vi "8FFTHanning窗校正子程序.vi"(6 "averaging parameters":T1={"averaging mode"=enum."No averaging", "weighting mode"=enum."Exponential", "number of averages"=10}, 7 "time signal":waveform(dbl) caption="时间信号") -> (0 "FFT幅值":cluster{"f0":dbl, "df":dbl, "magnitude":dbl[]}(graph), 2 "FFT相位":cluster{"f0":dbl, "df":dbl, "phase":dbl[]}(graph), 3 "频率":dbl)   [LabVIEW 2017]
uses:
  <vilib>/Analysis/4window.llb/windowTd.ctl
  <vilib>/measure/maspectr.llb/FFT Spectrum (Mag-Phase) for 1 Chan.vi
  <vilib>/measure/NI_MAPro.lvlib
  <vilib>/Analysis/NI_AALPro.lvlib
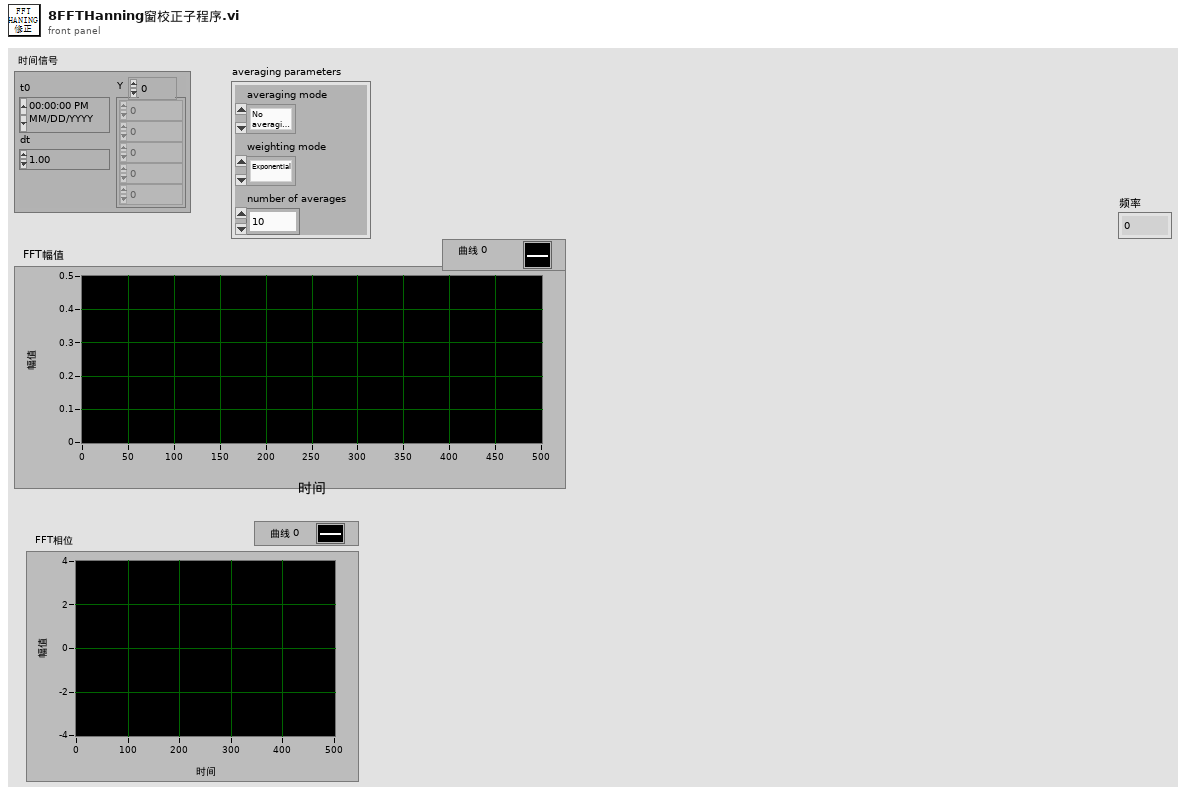
[diagram p1: front panel]
types:
  T1 = cluster{"averaging mode":enum16{"No averaging", "Vector averaging", "RMS averaging", "Peak hold"}, "weighting mode":enum16{"Linear", "Exponential"}, "number of averages":u32}
  T2 = typedef "NI_AALPro.lvlib/windowTd.ctl" = u32
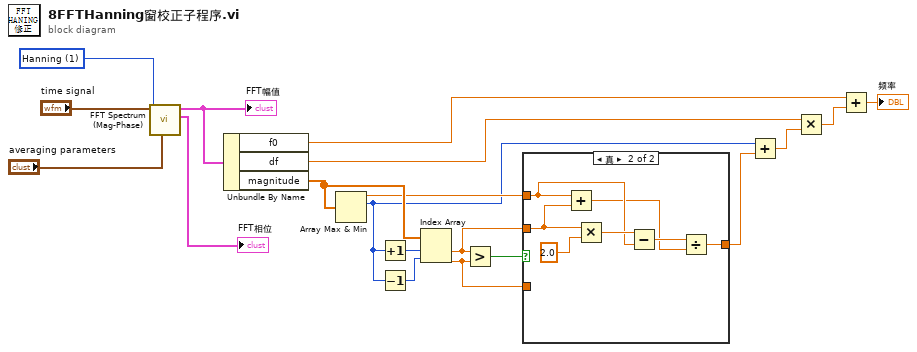
[diagram p0: block diagram]
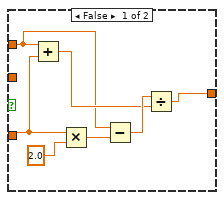
[diagram p2: hidden frame]
diagram:
  w17 = T2 1 items=["矩形"=0, "Hanning"=1, "Hamming"=2, "Blackman-Harris"=3, "Exact Blackman"=4, "Blackman"=5, "Flat Top"=6, "4阶Blackman-Harris "=7, "7阶Blackman-Harris"=8, "Low Sidelobe"=9, "Blackman Nuttall"=11, "三角"=30, "Bartlett-Hanning"=31, "Bohman"=32, "Parzen"=33, "Welch"=34, "Kaiser"=60, "Dolph-Chebyshev"=61, "高斯"=62] ("window")
  n1 = call-poly <vilib>:"FFT Spectrum (Mag-Phase).vi"("averaging parameters"="averaging parameters", "window"=w17, "time signal"="time signal") -> ("phase"=→"FFT相位":cluster{"f0":dbl, "df":dbl, "phase":dbl[]}, "magnitude"=w19:cluster{"f0":dbl, "df":dbl, "magnitude":dbl[]})  [unwired: 4 in, 3 out]
  "FFT幅值" <- w19
  n2 = Unbundle By Name(w19) -> ("f0"=w14:dbl, "df"=w12:dbl, "magnitude"=w8:dbl[])
  n3 = Array Max & Min(array=w8) -> (max value=w3:dbl, max index (indices)=w1:i32)  [unwired: 2 out]
  n4 = Increment(x=w1) -> (x+1=w13:i32)
  n5 = Decrement(x=w1) -> (x-1=w7:i32)
  n6 = Index Array(array=w8, index #1=w13, index #2=w7) -> (element #1=w5:dbl, element #2=w4:dbl)
  n7 = Greater?(x=w5, y=w4) -> (0:w6:bool)
  n8 = case shown="真" w6 {
    tunnel: w5 -> [_ w32]
    tunnel: w4 -> [w21 _]
    tunnel: w3 -> [w23 w30]
    tunnel: [w20 w27] -> w2
    frame False {
      n9 = Add(x=w23, y=w21) -> (x+y=w24:dbl)
      n10 = Multiply(x=w21, y=2.0) -> (x*y=w22:dbl)
      n11 = Subtract(x=w23, y=w22) -> (x-y=w25:dbl)
      n12 = Divide(x=w25, y=w24) -> (x/y=w20:dbl)
    }
    frame True {
      n13 = Add(x=w30, y=w32) -> (x+y=w28:dbl)
      n14 = Multiply(x=w32, y=2.0) -> (x*y=w31:dbl)
      n15 = Subtract(x=w31, y=w30) -> (x-y=w29:dbl)
      n16 = Divide(x=w29, y=w28) -> (x/y=w27:dbl)
    }
  }
  n17 = Add(x=w1, y=w2) -> (x+y=w11:dbl)
  n18 = Multiply(x=w12, y=w11) -> (x*y=w9:dbl)
  n19 = Add(x=w14, y=w9) -> (x+y=→"频率":dbl)
